vi "Get Display Name for Cfg file.vi"(8 "error in (no error)":errorcluster, 11 "file path":path) -> (0 "error out":errorcluster, 3 "display string":string)   [LabVIEW 2022 SP3, in "Config Dialog.lvlib"]
uses:
  Config Dialog.lvlib
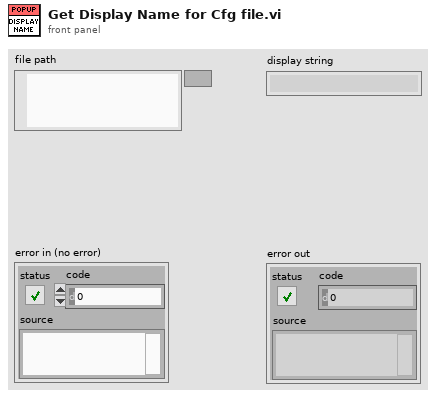
[diagram p1: front panel]
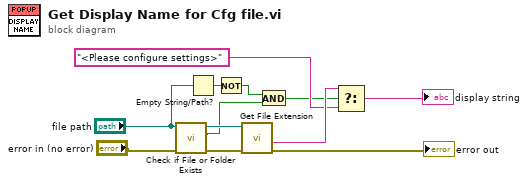
[diagram p0: block diagram]
diagram:
  n1 = call <vilib>:"Check if File or Folder Exists.vi"("error in (no error)"="error in (no error)", "path"="file path") -> ("error out"=w9:errorcluster, "file or folder exists?"=w4:bool, "dup path"=w8:path)  [unwired: 7 in]
  n2 = Empty String/Path?(string/path="file path") -> (empty?=w5:bool)
  n3 = Not(x=w5) -> (.not. x?=w3:bool)
  n4 = call <vilib>:"Get File Extension.vi"("error in (no error)"=w9, "file"=w8) -> ("error out"=→"error out":errorcluster, "filename without extension"=w7:string)  [unwired: 5 in, 3 out]
  n5 = And(x=w3, y=w4) -> (x .and. y?=w2:bool)
  n6 = Select(t=w7, s=w2, f="<Please configure settings>" ("t")) -> (s? t:f=→"display string":string)
